vi "odor config arr color update (sub-vi).vi"(8 "error in (no error)":errorcluster, 11 "array refnum":refnum<vi>) -> (0 "error out":errorcluster, 3 "array refnum out":refnum<vi>)   [LabVIEW 2021]
uses:
  type-defs/odor color enum (type def).ctl
  type-defs/odor color (type def).ctl
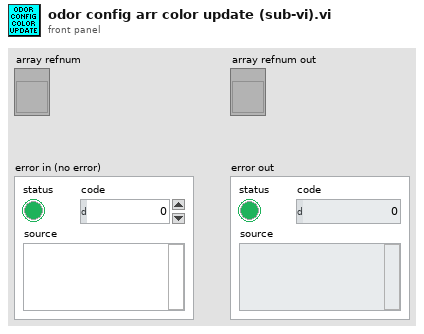
[diagram p1: front panel]
types:
  T1 = typedef "odor color (type def).ctl" = u16
  T2 = typedef "odor color enum (type def).ctl" = enum16{"white", "blue", "red", "orange", "yellow", "green", "magenta", "brown", "black", "[none]"}
  T3 = typedef "odor description array (type def).ctl" = T4[]
  T4 = typedef "odor info cluster (type def).ctl" = cluster{"odor channel":T5, "odor description":string, "odor color":T1, "odor channel active":bool}
  T5 = typedef "odor selection (type def).ctl" = enum16{"[none]", "odor 1", "odor 2", "odor 3", "odor 4", "odor 5", "odor 6", "odor 7", "odor 8", "odor 9", "odor 10"}
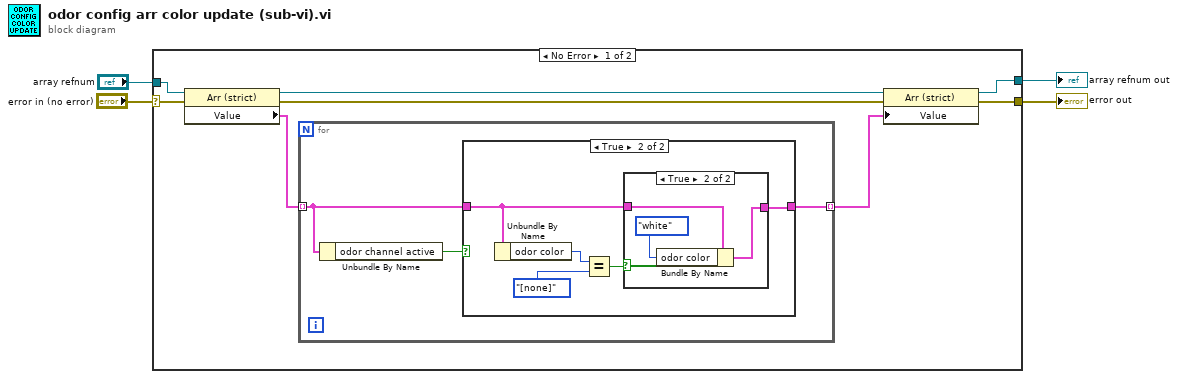
[diagram p0: block diagram]
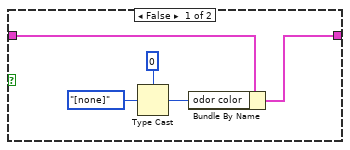
[diagram p2: hidden frame]
diagram:
  n1 = case shown="No Error" "error in (no error)" {
    selector: "error in (no error)" -> [w7 w30]
    tunnel: [w12 w30] -> w4
    tunnel: "array refnum" -> [w6 w31]
    tunnel: [w5 w31] -> w1
    frame No Error {
      n2 = property class="Arr (strict)"(reference=w6, error in=w7) -> (reference out=w11:refnum<vi>, error out=w10:errorcluster, "Value"=w8:T3)
      n3 = for {
        tunnel: w8 -> [w14] mode=indexing
        tunnel: [w13] -> w9 mode=indexing
        n4 = Unbundle By Name(w14) -> ("odor channel active"=w15:bool)
        n5 = case shown="True" w15 {
          tunnel: [w16 w21] -> w13
          tunnel: w14 -> [w20 w22]
          frame False {
            n6 = Type Cast(type=T1 0 ("odor color"), x=odor_color_enum_(type_def)."[none]" ("Enum")) -> (*(type *) &x=w17:T1)
            n7 = Bundle By Name(cluster=w20, "odor color"=w17) -> (w16:T4)
          }
          frame True {
            n8 = Unbundle By Name(w22) -> ("odor color"=w25:T1)
            n9 = Equal?(x=w25, y=odor_color_enum_(type_def)."[none]" ("Enum")) -> (x = y?=w23:bool)
            n10 = case shown="True" w23 {
              tunnel: w22 -> [w26 w29]
              tunnel: [w26 w28] -> w21
              frame False {
              }
              frame True {
                n11 = Bundle By Name(cluster=w29, "odor color"=odor_color_enum_(type_def)."white" ("Enum")) -> (w28:T4)
              }
            }
          }
        }
      }
      n12 = property class="Arr (strict)"(reference=w11, error in=w10, "Value"=w9) -> (reference out=w5:refnum<vi>, error out=w12:errorcluster)
    }
    frame Error {
    }
  }
  "array refnum out" <- w1
  "error out" <- w4
